vi "calc_omega.vi"(0 "OldNc":i64, 1 "prev_omega":dbl, 2 "MaxDeltaNc":i64, 3 "MaxNc":i64, 4 "M":dbl, 5 "error in (no error)":errorcluster) -> (6 "omega":dbl, 7 "Nc":i64, 8 "error out":errorcluster)   [LabVIEW 2021]
uses:
  ISRglobals.vi
  <vilib>/Analysis/NI_AALBase.lvlib
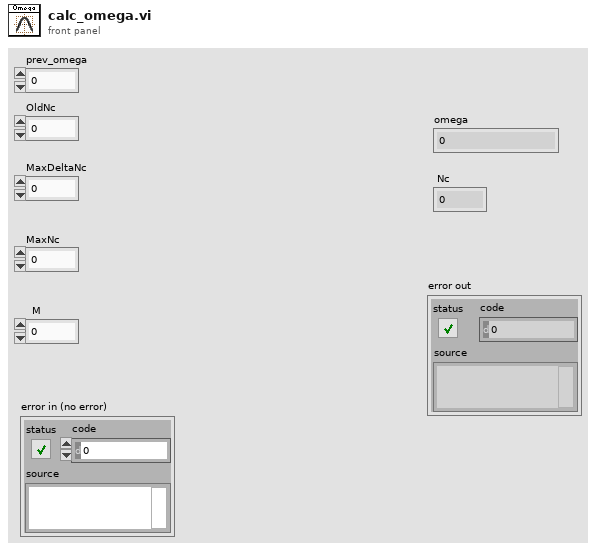
[diagram p1: front panel]
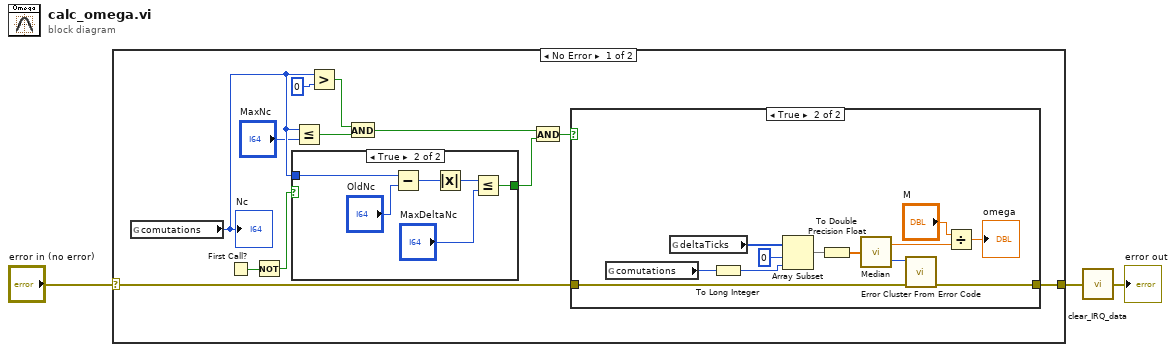
[diagram p0: block diagram]
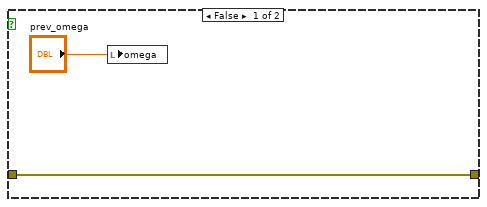
[diagram p2: hidden frame]
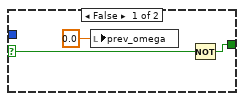
[diagram p3: hidden frame]
diagram:
  n1 = case shown="No Error" "error in (no error)" {
    selector: "error in (no error)" -> [w8 w39]
    tunnel: [w9 w39] -> w2
    frame No Error {
      n2 = global read "ISRglobals.vi" "comutations"() -> (w5:i64)
      "Nc" <- w5
      n3 = First Call?() -> (First Call?: T/F=w12:bool)
      n4 = Not(x=w12) -> (.not. x?=w11:bool)
      n5 = case shown="True" w11 {
        selector: w11 -> [w32 _]
        tunnel: w5 -> [_ w38]
        tunnel: [w31 w37] -> w6
        frame False {
          n6 = local write "prev_omega"(0.0 ("OldRPM")) -> ()
          n7 = Not(x=w32) -> (.not. x?=w31:bool)
        }
        frame True {
          n8 = Subtract(x=w38, y="OldNc") -> (x-y=w35:i64)
          n9 = Absolute Value(x=w35) -> (abs(x)=w36:i64)
          n10 = Less Or Equal?(x=w36, y="MaxDeltaNc") -> (x <= y?=w37:bool)
        }
      }
      n11 = Less Or Equal?(x=w5, y="MaxNc") -> (x <= y?=w7:bool)
      n12 = Greater?(x=w5, y=i64 0) -> (0:w14:bool)
      n13 = And(x=w14, y=w7) -> (x .and. y?=w13:bool)
      n14 = And(x=w13, y=w6) -> (x .and. y?=w10:bool)
      n15 = case shown="True" w10 {
        tunnel: w8 -> [w17 w24]
        tunnel: [w17 w22] -> w9
        frame False {
          n16 = local write "omega"("prev_omega") -> ()
        }
        frame True {
          n17 = global read "ISRglobals.vi" "comutations"() -> (w20:i64)
          n18 = global read "ISRglobals.vi" "deltaTicks"() -> (w19:i64[])
          n19 = To Long Integer(number=w20) -> (32bit integer=w21:i32)
          n20 = Array Subset(array=w19, index=0, length=w21) -> (w28:i64[])
          n21 = To Double Precision Float(number=w28) -> (double precision float=w27:dbl[])
          n22 = call <vilib>:"Median.vi"("X"=w27) -> ("median"=w25:dbl, "error"=w23:i32)
          n23 = call <vilib>:"Error Cluster From Error Code.vi"("error in (no error)"=w24, "error code (0)"=w23) -> ("error out"=w22:errorcluster)  [unwired: 7 in]
          n24 = Divide(x="M", y=w25) -> (x/y=→"omega":dbl)
        }
      }
    }
    frame Error {
    }
  }
  n25 = call "clear_IRQ_data.vi"("error IO"=w2) -> ("error IO 2"=→"error out":errorcluster)
